vi "servor rpm test.vi"() -> ()   [LabVIEW 2018]
uses:
  <vilib>/Platform/TimedLoop/XDataNode/timing_clust.ctl
  <vilib>/Platform/TimedLoop/XDataNode/nitl_modes.ctl
  <vilib>/Platform/TimedLoop/XDataNode/wakeup.ctl
  <vilib>/FPGAPlugInAG/myRIO-1900/niLvFpga_Open_myRIO-1900.vi
  <vilib>/rvi/interface/common/dynamic/niFpgaDynamicAddResources.vi
  <vilib>/Utility/error.llb/Error Cluster From Error Code.vi
  <vilib>/rvi/errors/niLvFpgaAdjustHostInterfaceError.vi
  <vilib>/rvi/interface/nirviOpenFPGA/nirviOpenFPGA.xnode
  FPGA Bitfiles/Dentalrobot_FPGATarget_FPGADentalroboto_PTkoih3chUc.lvbitx
  FPGA/FPGA_myRIO.vi
  <vilib>/rvi/interface/nirviReadWriteControl/nirviReadWriteControl.xnode
  <vilib>/Platform/TimedLoop/XDataNode/XDataNode.xnode
  <vilib>/Platform/TimedLoop/XDataNode/XDNodeRunTimeDep.lvlib
  <vilib>/rvi/interface/Simulation/niFpgaSimulationCallBeginRW.vi
  NiFpgaLv.dll
panel:
  in  "Counts/revolution":i32=34304
  out "JumpBy2Error 4":i16
  out "Waveform Chart":dbl(graph)
  in  "stop":bool
  out "Position4":i32
  in  "Reset 4":bool
  in  "DC":fxp<+,32,0>
  in  "DIR4":bool
  in  "ENA4":bool
  out "finished late":dbl
  # "275:1   140800\n67:1      34304"
  # "rpm"
  # "275:1"
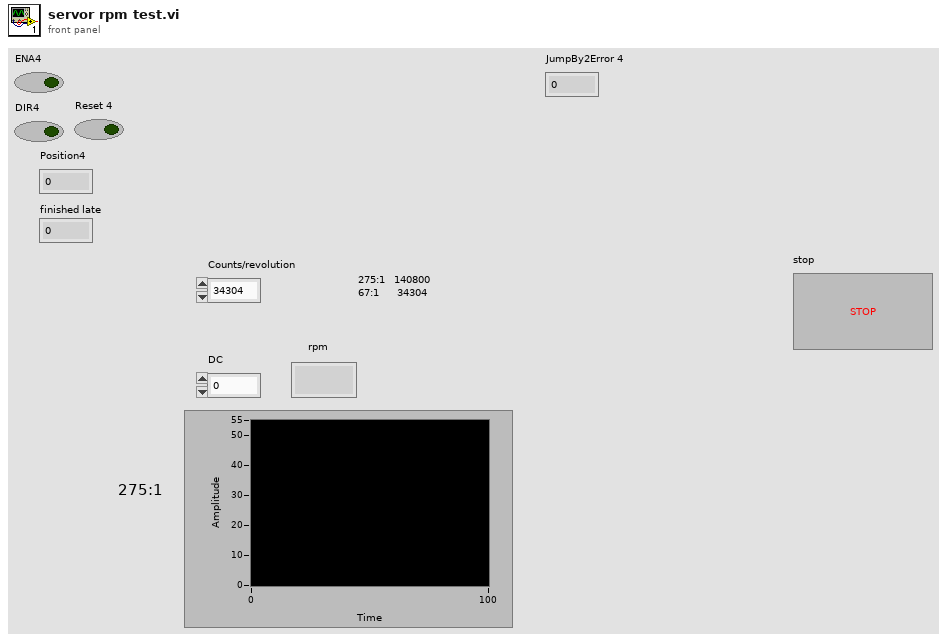
[diagram p1: front panel]
types:
  T1 = typedef "XDNodeRunTimeDep.lvlib/timing_clust.ctl" = cluster{"Expected End [f-1]":u64, "Actual End [f-1]":u64, "Finished Late? [f-1]":bool, "Expected End [i-1]":u64, "Actual End [i-1]":u64, "Finished Late? [i-1]":bool, "Expected Start [i]":u64, "Actual Start [i]":u64, "Expected Start [f]":u64, "Actual Start [f]":u64, "Source Name":string, "Structure Name":string, "Period":i64, "Deadline":i64, "Offset":i64, "Start":i64, "Priority":i32, "Timeout":i32, "Mode":T2, "Wakeup Reason":T3, "Error":errorcluster, "Source Type":string, "Secondary Source Type":string, "Global End Time":u64, "Global Start Time":u64, "Frame Duration":u64, "Iteration Duration":u64, "Assigned CPU":i32, "I/O Scan Engine Mode":u32}
  T2 = typedef "XDNodeRunTimeDep.lvlib/nitl_modes.ctl" = enum32{"No Change", "Process missed periods, maintain original phase", "Discard missed periods, maintain original phase", "Process missed periods, ignore original phase", "Discard missed periods, ignore original phase"}
  T3 = typedef "XDNodeRunTimeDep.lvlib/wakeup.ctl" = enum32{"Normal", "Aborted", "Asynchronous wakeup", "Timing source error", "Timed loop error", "Timeout"}
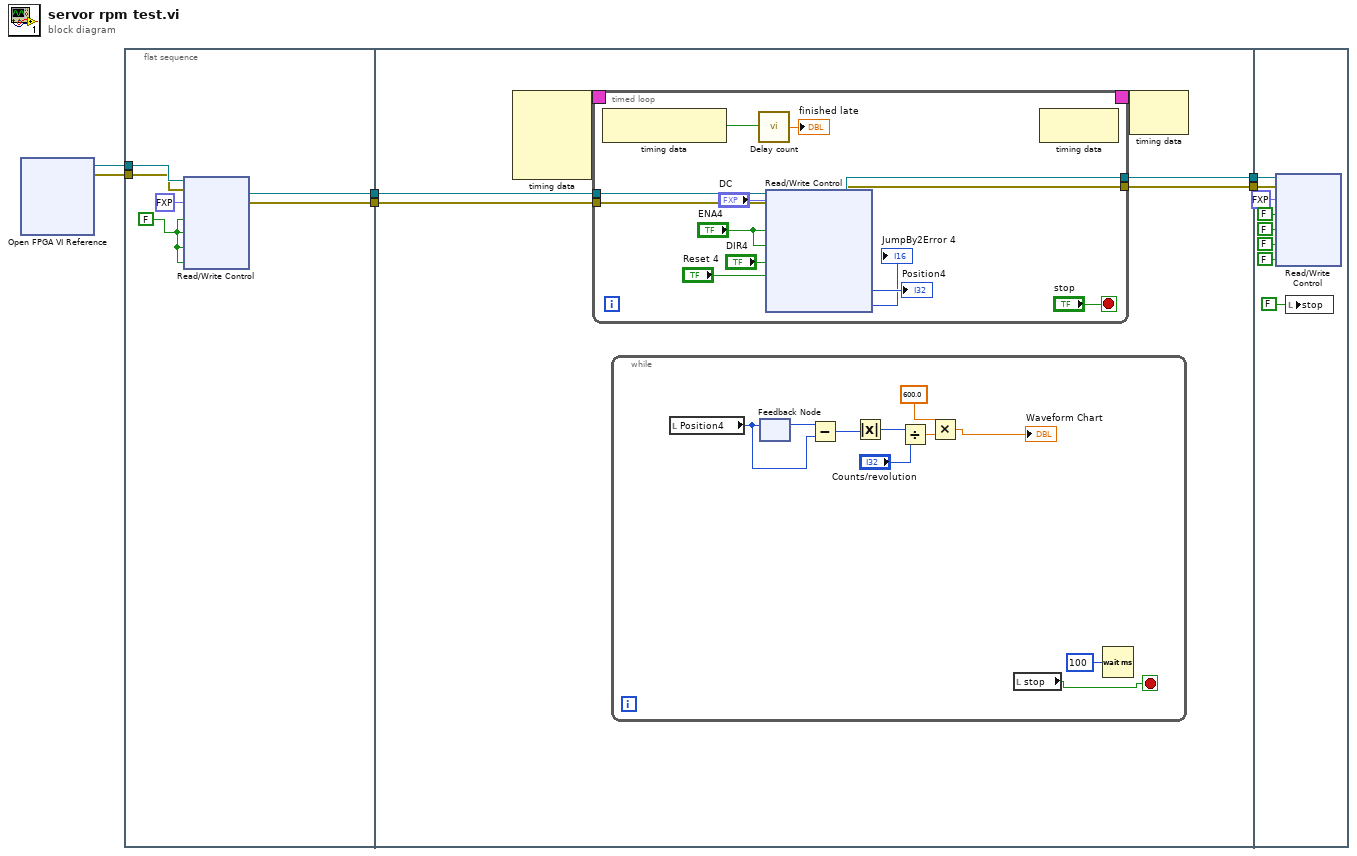
[diagram p0: block diagram]
diagram:
  n1 = xnode "Open FPGA VI Reference"() -> ("FPGA VI Reference Out"=w6:refnum<k20>, "error out"=w5:errorcluster)  [unwired: 2 in]
  n2 = flat-sequence {
    tunnel: w6 -> [w12]
    tunnel: w5 -> [w11]
    tunnel: [w8] -> w4
    tunnel: [w7] -> w3
    tunnel: w4 -> [w16]
    tunnel: w3 -> [w15]
    tunnel: [w14] -> w2
    tunnel: [w13] -> w1
    tunnel: w2 -> [w54]
    tunnel: w1 -> [w53]
    frame #0 {
      w10 = FALSE
      n3 = xnode "Read/Write Control"("FPGA VI Reference In"=w12, "error in"=w11, "CH4 DC"=fxp<+,32,0> 0.0, "ENA4"=w10, "STBY4"=w10, "DIR4"=w10, "Reset 4"=w10) -> ("FPGA VI Reference Out"=w8:refnum<k20>, "error out"=w7:errorcluster)
    }
    frame #1 {
      n4 = node-c288() -> (w18:T1)  [unwired: 4 in]
      n5 = timed-loop {
        timing: w18 -> [_]
        timing-out: [_] -> w17
        tunnel: w16 -> [w41]
        tunnel: w15 -> [w40]
        tunnel: [w39] -> w14
        tunnel: [w38] -> w13
        stop <- "stop" stop-if-true
        n6 = node-c288() -> (w37:bool)  [unwired: 1 in]
        n7 = call "Delay count.vi"("Finished Late? [i-1]"=w37) -> ("Count"=→"finished late":dbl)
        n8 = xnode "Read/Write Control"("FPGA VI Reference In"=w41, "error in"=w40, "CH4 DC"="DC", "ENA4"="ENA4", "STBY4"="ENA4", "DIR4"="DIR4", "Reset 4"="Reset 4") -> ("FPGA VI Reference Out"=w39:refnum<k20>, "error out"=w38:errorcluster, "Position4"=→"Position4":i32, "JumpBy2Error 4"=→"JumpBy2Error 4":i16)
        n9 = node-c288() -> ()  [unwired: 1 in, 1 out]
      }
      n10 = while {
        stop <- w21 stop-if-true
        n11 = local read "Position4"() -> (w27:i32)
        n12 = feedback-in #1(w27) -> ()
        n13 = feedback #1() -> (w28:i32)  [unwired: 1 in]
        n14 = Subtract(x=w28, y=w27) -> (x-y=w26:i32)
        n15 = Absolute Value(x=w26) -> (abs(x)=w25:i32)
        n16 = Divide(x=w25, y="Counts/revolution") -> (x/y=w24:dbl)
        n17 = Multiply(x=600.0, y=w24) -> (x*y=→"Waveform Chart":dbl)
        n18 = local read "stop"() -> (w21:bool)
        n19 = Wait (ms)(milliseconds to wait=u32 100) -> ()  [unwired: 1 out]
      }
      n20 = node-c288(w17) -> ()  [unwired: 1 out]
    }
    frame #2 {
      n21 = xnode "Read/Write Control"("FPGA VI Reference In"=w54, "error in"=w53, "CH4 DC"=fxp<+,32,0> 0.0, "ENA4"=FALSE, "STBY4"=FALSE, "DIR4"=FALSE, "Reset 4"=FALSE) -> ()  [unwired: 2 out]
      n22 = local write "stop"(FALSE ("stop")) -> ()
    }
  }
